vi "Read Temp Units.vi"(8 "error in (no error)":errorcluster, 11 "F4T in":refnum<class "F4T.lvclass">) -> (0 "error out":errorcluster, 2 "Temp Units":T1, 3 "F4T out":refnum<class "F4T.lvclass">)   [LabVIEW 2018, in "F4T.lvlib" / "F4T.lvclass"]
uses:
  F4T.lvclass
  Custom Controls/Temp Units.ctl
  F4T.lvclass/F4T.ctl
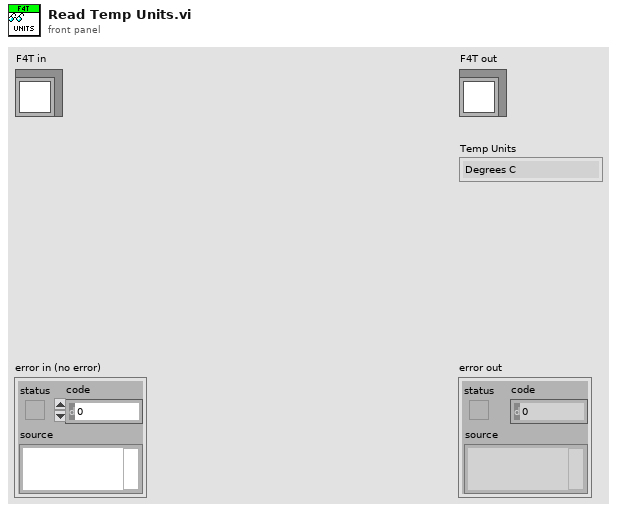
[diagram p1: front panel]
types:
  T1 = typedef "F4T.lvlib/F4T.lvclass/Temp Units.ctl" = enum16{"Degrees C", "Degrees F"}
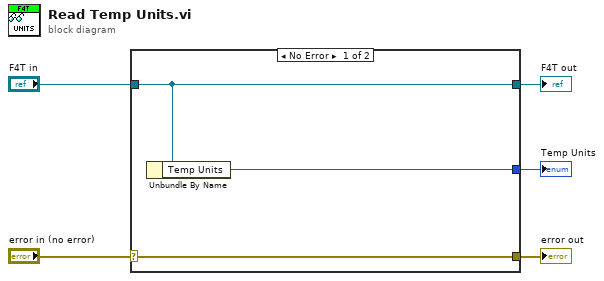
[diagram p0: block diagram]
diagram:
  n1 = case shown="No Error" "error in (no error)" {
    selector: "error in (no error)" -> [w8 w9]
    tunnel: [w8 w9] -> w4
    tunnel: [w7 w10] -> w2
    tunnel: "F4T in" -> [w7 w10]
    tunnel: [w6 _] -> w1
    frame No Error {
      n2 = Unbundle By Name(w7) -> ("Temp Units"=w6:T1)
    }
    frame Error {
    }
  }
  "error out" <- w4
  "F4T out" <- w2
  "Temp Units" <- w1
